vi "Warning.vi"() -> ()   [LabVIEW 2017, in "Assertions.Tests.lvlib" / "Assert Error.lvlib"]
uses:
  Assert Error.lvlib
  src/Transparent Assertions/Assertions/Assertions.lvlib
panel:
  out "error out":errorcluster
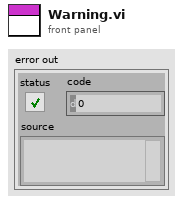
[diagram p1: front panel]
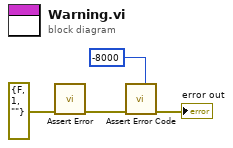
[diagram p0: block diagram]
diagram:
  n1 = call "Assert Error.vi"("error in (no error)"=errorcluster {"status"=FALSE, "code"=1, "source"=""}) -> ("error out"=w3:errorcluster)  [unwired: 10 in]
  n2 = call "Assert Error Code.vi"("Expected"=-8000, "error in (no error)"=w3) -> ("error out"=→"error out":errorcluster)  [unwired: 9 in]
